vi "Multicolumn_Listbox_Get selected row strings.vi"(8 "error in (no error)":errorcluster, 11 "MulticolumnListbox in":refnum<vi>) -> (0 "error out":errorcluster, 2 "Selected row strings":string[](array[string]), 3 "MulticolumnListbox out":refnum<vi>)   [LabVIEW 2013]
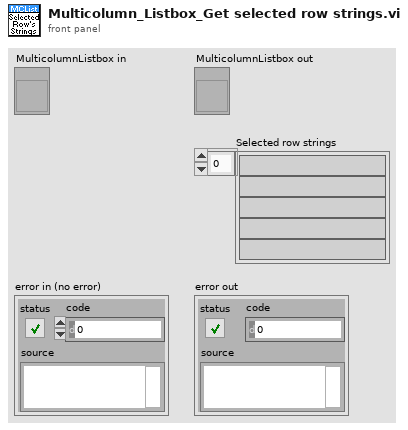
[diagram p1: front panel]
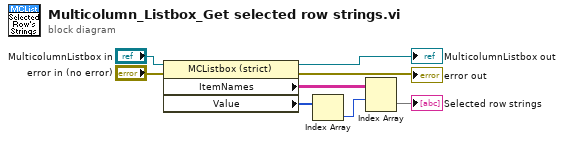
[diagram p0: block diagram]
diagram:
  n1 = property on="Property Node" class="MCListbox (strict)"(reference="MulticolumnListbox in", error in="error in (no error)") -> (reference out=→"MulticolumnListbox out":refnum<vi>, error out=→"error out":errorcluster, "ItemNames"=w5:string[][], "Value"=w4:i32[])
  n2 = Index Array(array=w4) -> (element=w6:i32)  [unwired: 1 in]
  n3 = Index Array(array=w5, index (row)=w6) -> (element=→"Selected row strings":string[])  [unwired: 1 in]
